vi "Configure Horizontal.vi"(8 "error in":errorcluster, 11 "Scope PXI Base CFG in":refnum<class "Scope PXI Base CFG.lvclass">) -> (0 "error out":errorcluster, 3 "Scope PXI Base CFG out":refnum<class "Scope PXI Base CFG.lvclass">)   [LabVIEW 2023, in "Scope PXI Base CFG.lvclass"]
uses:
  Scope PXI Base CFG.lvclass
  Scope PXI Base CFG.lvclass/Scope PXI Base CFG.ctl
  <vilib>/Utility/error.llb/Error Cluster From Error Code.vi
  <vilib>/ErrorRing/Error Ring.xnode
  Configuration JSON Base/CFG JSON Base.lvclass
  2e7921dc-a2d8-456a-8bcd-efe2ea717c44.vi
  D:/git/HAL/HAL GOOP4/Scope/Scope Base CFG/Scope Base CFG.lvclass
  D:/git/HAL/HAL GOOP4/Configuration JSON Base/CFG JSON Base.lvclass
  D:/git/HAL/HAL GOOP4/Interfaces/IConfigure/IConfigure.lvclass
  D:/git/HAL/HAL GOOP4/Scope/Scope PXI/Base CFG/Scope PXI Base CFG.lvclass
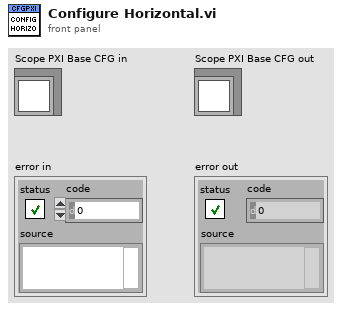
[diagram p1: front panel]
types:
  T1 = cluster{"Enforce Realtime":bool, "Number of Records":i32, "Min Sample Rate":dbl, "Reference Position":dbl, "Min Record Length":i32}
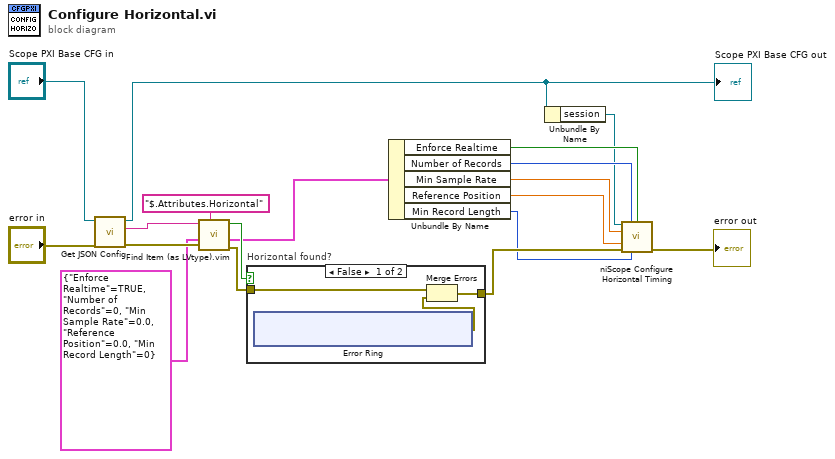
[diagram p0: block diagram]
diagram:
  n1 = call "Get JSON Config.vi"("error in (no error)"="error in", "CFG Base in"="Scope PXI Base CFG in") -> ("error out"=w16:errorcluster, "<JSON>Config>"=w15:string, "CFG Base out"=w2:refnum<class "Scope PXI Base CFG.lvclass">)  [unwired: 7 in]
  "Scope PXI Base CFG out" <- w2
  n2 = call "Find Item (as LVtype).vim"("$Path or Item Name"="$.Attributes.Horizontal", "error in (no error)"=w16, "Data Type and Default Value"=T1 {"Enforce Realtime"=TRUE, "Number of Records"=0, "Min Sample Rate"=0.0, "Reference Position"=0.0, "Min Record Length"=0}, "JSON"=w15) -> ("error out"=w13:errorcluster, "Data"=w8:T1, "Found"=w12:bool)  [unwired: 4 in, 1 out]
  n3 = case "Horizontal found?" shown="False" w12 {
    tunnel: [w21 w27] -> w10
    tunnel: w13 -> [w19 w27]
    frame False {
      n4 = xnode "Error Ring"() -> ("error out"=w20:errorcluster)
      n5 = Merge Errors(w19, w20) -> (w21:errorcluster)
    }
    frame True {
    }
  }
  n6 = Unbundle By Name(w8) -> ("Enforce Realtime"=w7:bool, "Number of Records"=w6:i32, "Min Sample Rate"=w5:dbl, "Reference Position"=w4:dbl, "Min Record Length"=w3:i32)
  n7 = Unbundle By Name(w2) -> ("session"=w1:refnum<k15>)
  n8 = call <instrlib>:"niScope Configure Horizontal Timing.vi"("instrument handle"=w1, "number of records"=w6, "enforce realtime"=w7, "min sample rate"=w5, "reference position"=w4, "error in"=w10, "min record length"=w3) -> ("error out"=→"error out":errorcluster)  [unwired: 7 in, 1 out]
